vi "Reverse Selection Symbol.vi"(8 "error in":errorcluster, 10 "Coords":T1, 11 "GU List Ref":refnum<vi>) -> (0 "error out":errorcluster, 2 "Selected GU":i32[](array[numeric]))   [LabVIEW 2020, in "GUCalibration2.lvlib"]
uses:
  GUCalibration2.lvlib
  <vilib>/Utility/miscctls.llb/LVPoint32TypeDef.ctl
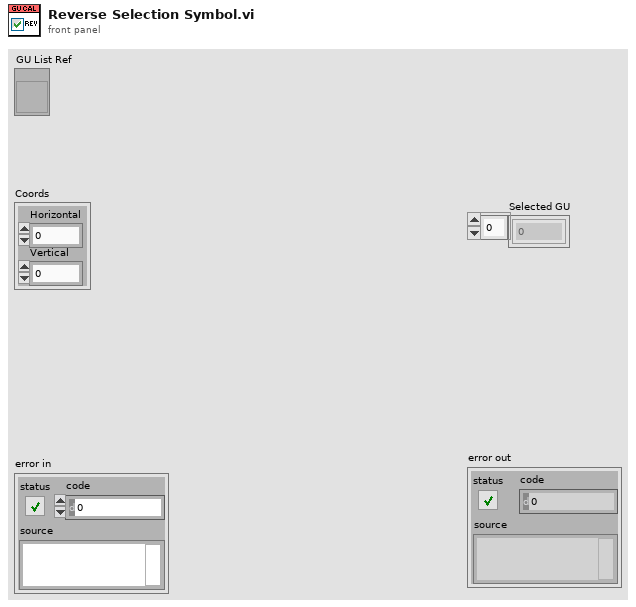
[diagram p1: front panel]
types:
  T1 = typedef "LVPoint32TypeDef.ctl" = cluster{"Horizontal":i32, "Vertical":i32}
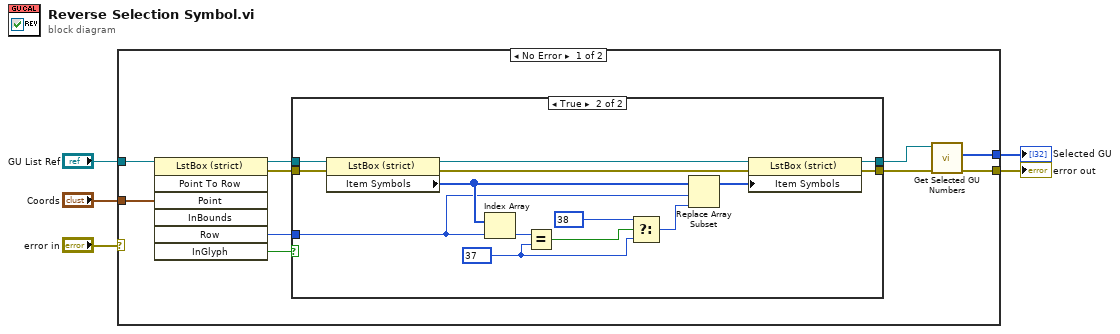
[diagram p0: block diagram]
diagram:
  n1 = case shown="No Error" "error in" {
    selector: "error in" -> [_ w32]
    tunnel: "GU List Ref" -> [w15 _]
    tunnel: "Coords" -> [w14 _]
    tunnel: [w7 w32] -> w3
    tunnel: [w6 _] -> w1
    frame No Error {
      n2 = invoke class="LstBox (strict)" method="Point To Row"(reference=w15, "Point"=w14) -> (reference out=w10:refnum<vi>, error out=w11:errorcluster, "Row"=w12:i32, "InGlyph"=w13:bool)  [unwired: 5 in, 3 out]
      n3 = case shown="True" w13 {
        tunnel: w12 -> [_ w24]
        tunnel: w11 -> [w17 w30]
        tunnel: w10 -> [w16 w31]
        tunnel: [w17 w21] -> w8
        tunnel: [w16 w18] -> w9
        frame False {
        }
        frame True {
          w27 = 37
          n4 = property class="LstBox (strict)"(reference=w31, error in=w30) -> (reference out=w22:refnum<vi>, error out=w23:errorcluster, "Item Symbols"=w29:i32[])
          n5 = Index Array(array=w29, index=w24) -> (element=w25:i32)
          n6 = Equal?(x=w25, y=w27) -> (x = y?=w28:bool)
          n7 = Select(t=38, s=w28, f=w27) -> (s? t:f=w26:i32)
          n8 = Replace Array Subset(array=w29, new element=w26, index=w24) -> (w19:i32[])
          n9 = property class="LstBox (strict)"(reference=w22, error in=w23, "Item Symbols"=w19) -> (reference out=w18:refnum<vi>, error out=w21:errorcluster)
        }
      }
      n10 = call "Get Selected GU Numbers.vi"("error in"=w8, "Listbox Refnum"=w9) -> ("error out"=w7:errorcluster, "Selected GU"=w6:i32[])  [unwired: 8 in]
    }
    frame Error {
    }
  }
  "error out" <- w3
  "Selected GU" <- w1
